vi "headVector.vi"(1 "vector":dbl[](array[numeric])) -> (0 "vector hat":T1)   [LabVIEW 2021]
uses:
  <vilib>/Analysis/Matrix/Datatypes/RealMatrix.ctl
  <vilib>/Analysis/Matrix/NI_Matrix.lvlib
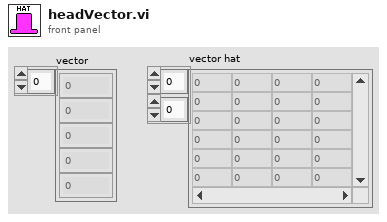
[diagram p1: front panel]
types:
  T1 = typedef "NI_Matrix.lvlib/RealMatrix.ctl" = dbl[][]
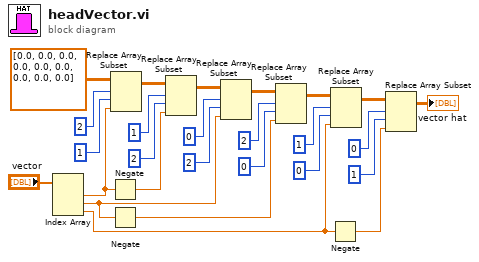
[diagram p0: block diagram]
diagram:
  n1 = Index Array(array="vector") -> (element #1=w7:dbl, element #2=w13:dbl, element #3=w16:dbl)  [unwired: 3 in]
  n2 = Negate(x=w7) -> (-x=w8:dbl)
  n3 = Negate(x=w13) -> (-x=w14:dbl)
  n4 = Replace Array Subset(array=T1 [[0.0, 0.0, 0.0], [0.0, 0.0, 0.0], [0.0, 0.0, 0.0]] ("matrix"), new element=w7, index (row)=2 ("disabled index (row)"), index (col)=1) -> (w4:T1)
  n5 = Replace Array Subset(array=w4, new element=w8, index (row)=1 ("disabled index (row)"), index (col)=2 ("disabled index (col)")) -> (w9:T1)
  n6 = Replace Array Subset(array=w9, new element=w13, index (row)=0 ("disabled index (row)"), index (col)=2) -> (w11:T1)
  n7 = Replace Array Subset(array=w11, new element=w14, index (row)=2 ("disabled index (row)"), index (col)=0 ("disabled index (col)")) -> (w15:T1)
  n8 = Negate(x=w16) -> (-x=w19:dbl)
  n9 = Replace Array Subset(array=w15, new element=w16, index (row)=1 ("disabled index (row)"), index (col)=0 ("disabled index (col)")) -> (w18:T1)
  n10 = Replace Array Subset(array=w18, new element=w19, index (row)=0 ("disabled index (row)"), index (col)=1) -> (→"vector hat":T1)
